vi "Labview0516326.vi"() -> ()   [LabVIEW 2015]
uses:
  <vilib>/Utility/miscctls.llb/LVDateTimeRec.ctl
panel:
  out "?":T1
  out "XY Graph":cluster{dbl[], dbl[]}[](graph)
  in  "stop 2":bool
  in  "alarm second":dbl
  in  "alarm minute":dbl
  in  "alarm hour":dbl
  in  "OK Button 3":bool
  in  "stop":bool
  in  "now time":bool
  in  "set se up":bool
  out "set second":dbl
  in  "set se down":bool
  in  "set min up":bool
  out "set minute":dbl
  in  "set  min down":bool
  in  "set hour up":bool
  in  "set hour down":bool
  out "set  hour":dbl
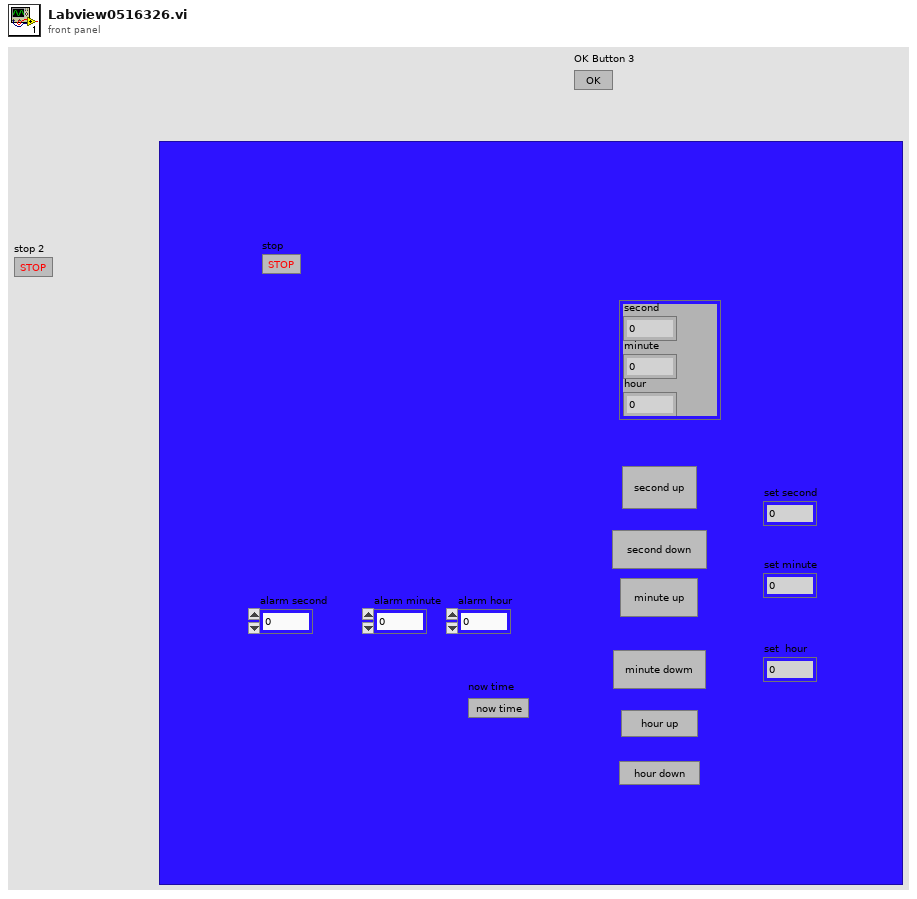
[diagram p1: front panel]
types:
  T1 = typedef "LVDateTimeRec.ctl" = cluster{"fractional second":dbl, "second":i32, "minute":i32, "hour":i32, "day of month":i32, "month":i32, "year":i32, "day of week":i32, "day of year":i32, "DST":i32}
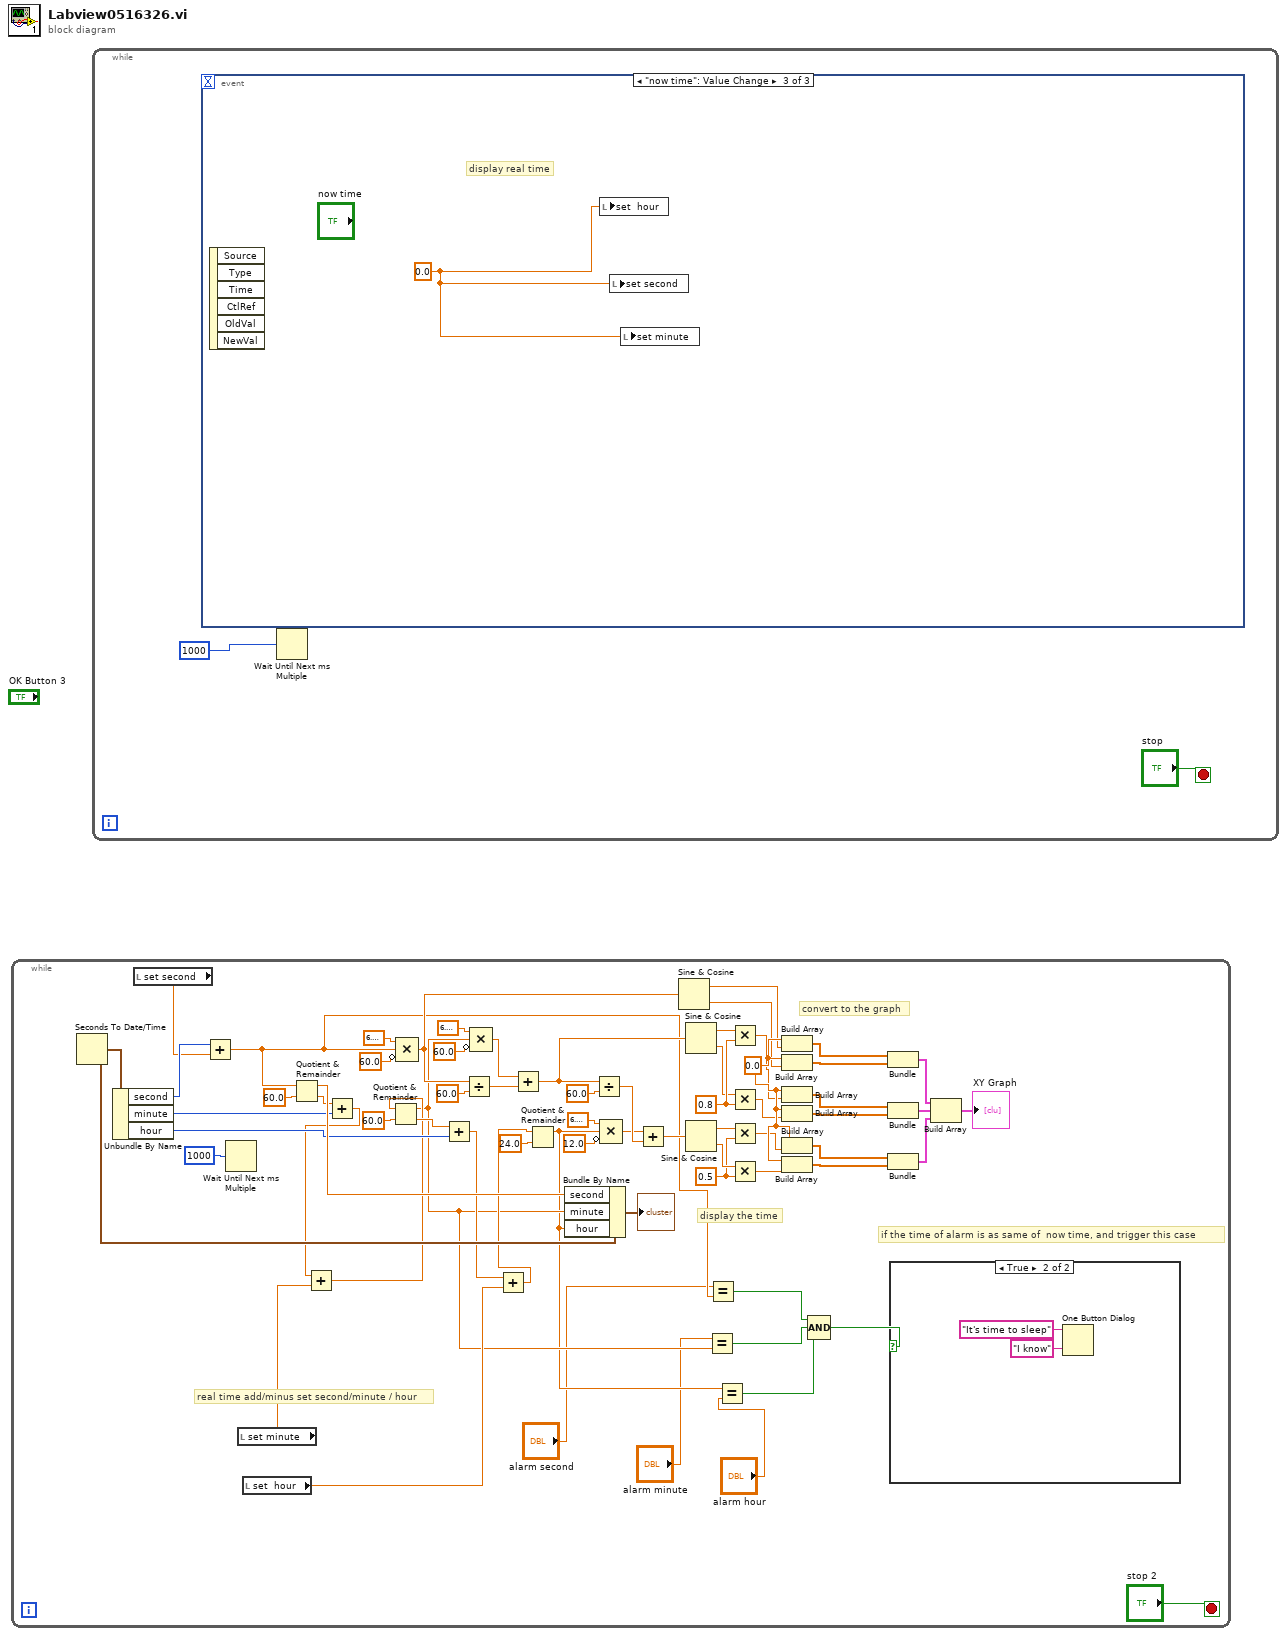
[diagram p0: block diagram]
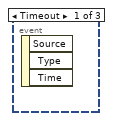
[diagram p3: hidden frame]
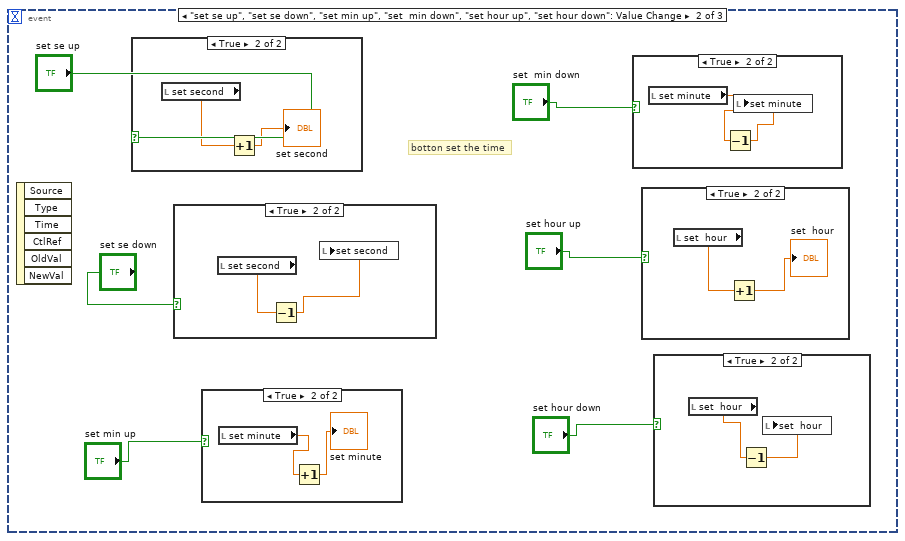
[diagram p4: hidden frame]
diagram:
  n1 = while {
    stop <- "stop 2" stop-if-true
    w47 = 0.0 ("Numeric")
    w48 = 0.5 ("Numeric")
    w53 = 0.8 ("Numeric")
    # "display the time"
    # "convert to the graph"
    # "real time add/minus set second/minute / hour"
    # "if the time of alarm is as same of  now time, and trigger this case"
    n2 = Seconds To Date/Time() -> (date time rec=w27:T1)  [unwired: 2 in]
    n3 = Unbundle By Name(w27) -> ("second"=w26:i32, "minute"=w22:i32, "hour"=w19:i32)
    n4 = local read "set second"() -> (w13:dbl)
    n5 = Add(x=w26, y=w13) -> (x+y=w10:dbl)
    n6 = Wait Until Next ms Multiple(millisecond multiple=u32 1000) -> ()  [unwired: 1 out]
    n7 = local read "set minute"() -> (w12:dbl)
    n8 = local read "set  hour"() -> (w11:dbl)
    n9 = Quotient & Remainder(x=w10, y=60.0) -> (x-y*floor(x/y)=w24:dbl, floor(x/y)=w23:dbl)
    n10 = Add(x=w23, y=w22) -> (x+y=w17:dbl)
    n11 = Add(x=w17, y=w12) -> (x+y=w16:dbl)
    n12 = Quotient & Remainder(x=w16, y=60.0) -> (x-y*floor(x/y)=w9:dbl, floor(x/y)=w18:dbl)
    n13 = Compound Arithmetic op=MULTIPLY(6.283185307179586, w10, invert 60.0 ("Numeric")) -> (w56:dbl)
    n14 = Add(x=w18, y=w19) -> (x+y=w15:dbl)
    n15 = Divide(x=w56, y=60.0) -> (x/y=w61:dbl)
    n16 = Compound Arithmetic op=MULTIPLY(6.283185307179586, w9, invert 60.0 ("Numeric")) -> (w60:dbl)
    n17 = Add(x=w15, y=w11) -> (x+y=w14:dbl)
    n18 = Add(x=w60, y=w61) -> (x+y=w55:dbl)
    n19 = Quotient & Remainder(x=w14, y=24.0) -> (x-y*floor(x/y)=w8:dbl)  [unwired: 1 out]
    n20 = Bundle By Name(cluster=w27, "second"=w24, "minute"=w9, "hour"=w8) -> (→"?":T1)
    n21 = Divide(x=w55, y=60.0) -> (x/y=w59:dbl)
    n22 = Compound Arithmetic op=MULTIPLY(6.283185307179586, w8, invert 12.0 ("Numeric")) -> (w57:dbl)
    n23 = Add(x=w57, y=w59) -> (x+y=w54:dbl)
    n24 = Sine & Cosine(0:w56) -> (1:w42:dbl, 2:w41:dbl)
    n25 = Sine & Cosine(0:w55) -> (1:w52:dbl, 2:w51:dbl)
    n26 = Sine & Cosine(0:w54) -> (1:w50:dbl, 2:w49:dbl)
    n27 = Equal?(x="alarm minute", y=w9) -> (x = y?=w3:bool)
    n28 = Equal?(x="alarm second", y=w10) -> (x = y?=w4:bool)
    n29 = Equal?(x=w8, y="alarm hour") -> (x = y?=w2:bool)
    n30 = Multiply(x=w52, y=w53) -> (x*y=w43:dbl)
    n31 = Multiply(x=w51, y=w53) -> (x*y=w44:dbl)
    n32 = Multiply(x=w50, y=w48) -> (x*y=w45:dbl)
    n33 = Multiply(x=w49, y=w48) -> (x*y=w46:dbl)
    n34 = Build Array(w47, w42) -> (w40:dbl[])
    n35 = Build Array(w47, w41) -> (w39:dbl[])
    n36 = Build Array(w47, w43) -> (w38:dbl[])
    n37 = Build Array(w47, w44) -> (w37:dbl[])
    n38 = Build Array(w47, w45) -> (w36:dbl[])
    n39 = Build Array(w47, w46) -> (w35:dbl[])
    n40 = Compound Arithmetic op=AND(w4, w3, w2) -> (w1:bool)
    n41 = Bundle(w40, w39) -> (w34:cluster{dbl[], dbl[]})  [unwired: 1 in]
    n42 = Bundle(w38, w37) -> (w33:cluster{dbl[], dbl[]})  [unwired: 1 in]
    n43 = Bundle(w36, w35) -> (w32:cluster{dbl[], dbl[]})  [unwired: 1 in]
    n44 = case shown="True" w1 {
      frame False {
      }
      frame True {
        n45 = One Button Dialog(message="It's time to sleep", button name ("OK")="I know") -> ()  [unwired: 1 out]
      }
    }
    n46 = Build Array(w34, w33, w32) -> (→"XY Graph":cluster{dbl[], dbl[]}[])
  }
  n47 = while {
    stop <- "stop" stop-if-true
    n48 = event shown="[2] \"now time\": Value Change" {
      selector: _ -> [_ _ _]
      dyn-events: _ -> [_ _ _]
      timeout: _ -> [_ _ _]
      event Timeout {
        n49 = event-data() -> ()  [unwired: 1 in, 3 out]
      }
      event "set se up", "set se down", "set min up", "set  min down", "set hour up", "set hour down": Value Change {
        # "botton set the time"
        n50 = event-data() -> ()  [unwired: 1 in, 6 out]
        n51 = case shown="True" "set se up" {
          frame False {
          }
          frame True {
            n52 = local read "set second"() -> (w90:dbl)
            n53 = Increment(x=w90) -> (x+1=→"set second":dbl)
          }
        }
        n54 = case shown="True" "set se down" {
          frame False {
          }
          frame True {
            n55 = local read "set second"() -> (w88:dbl)
            n56 = Decrement(x=w88) -> (x-1=w87:dbl)
            n57 = local write "set second"(w87) -> ()
          }
        }
        n58 = case shown="True" "set min up" {
          frame False {
          }
          frame True {
            n59 = local read "set minute"() -> (w85:dbl)
            n60 = Increment(x=w85) -> (x+1=→"set minute":dbl)
          }
        }
        n61 = case shown="True" "set  min down" {
          frame False {
          }
          frame True {
            n62 = local read "set minute"() -> (w84:dbl)
            n63 = Decrement(x=w84) -> (x-1=w83:dbl)
            n64 = local write "set minute"(w83) -> ()
          }
        }
        n65 = case shown="True" "set hour up" {
          frame False {
          }
          frame True {
            n66 = local read "set  hour"() -> (w82:dbl)
            n67 = Increment(x=w82) -> (x+1=→"set  hour":dbl)
          }
        }
        n68 = case shown="True" "set hour down" {
          frame False {
          }
          frame True {
            n69 = local read "set  hour"() -> (w80:dbl)
            n70 = Decrement(x=w80) -> (x-1=w79:dbl)
            n71 = local write "set  hour"(w79) -> ()
          }
        }
      }
      event "now time": Value Change {
        w91 = 0.0 ("Numeric")
        # "display real time"
        n72 = event-data() -> ()  [unwired: 1 in, 6 out]
        n73 = local write "set  hour"(w91) -> ()
        n74 = local write "set second"(w91) -> ()
        n75 = local write "set minute"(w91) -> ()
      }
    }
    n76 = Wait Until Next ms Multiple(millisecond multiple=u32 1000) -> ()  [unwired: 1 out]
  }
